vi "Read Statistics.vi"(6 "Maximum Time (10000 ms)":u32=10000, 7 "Data Source (0: Data Trace)":u16(ring) items=["Data Trace", "Memory Trace"], 8 "error in (no error)":errorcluster, 9 "Select Trace (1: 1)":u16(ring)=1 items=["1"=1, "2"=2, "3"=3, "4"=4, "5"=5, "6"=6, "7"=7, "8"=8], 10 "Measurement Type (6: Phase Noise)":u16(ring)=6 items=["AM Noise"=1, "Baseband Noise"=2, "Freq/Power"=3, "Spectrum"=4, "Transient"=5, "Phase Noise"=6, "User"=7], 11 "VISA resource name":refnum<visa-resource-name>) -> (0 "error out":errorcluster, 1 "Peak To Peak":dbl format="%^#_9g", 2 "Standard Deviation":dbl format="%^#_9g", 3 "VISA resource name out":refnum<visa-resource-name>, 5 "Mean":dbl format="%^#_9g")   [LabVIEW 2011, in "Agilent E5052X.lvlib"]
doc: "Reads the Mean, Standard Deviation and Peak To Peak values of either data or memory trace measurements of any measurement."
uses:
  Agilent E5052X.lvlib
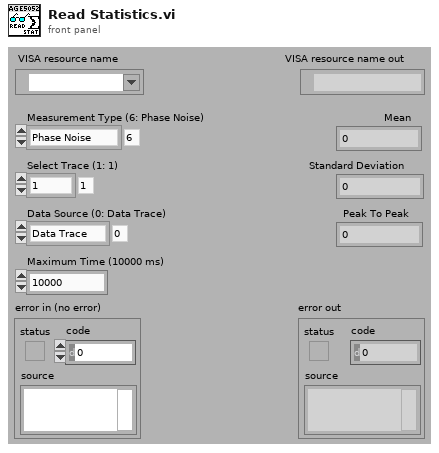
[diagram p1: front panel]
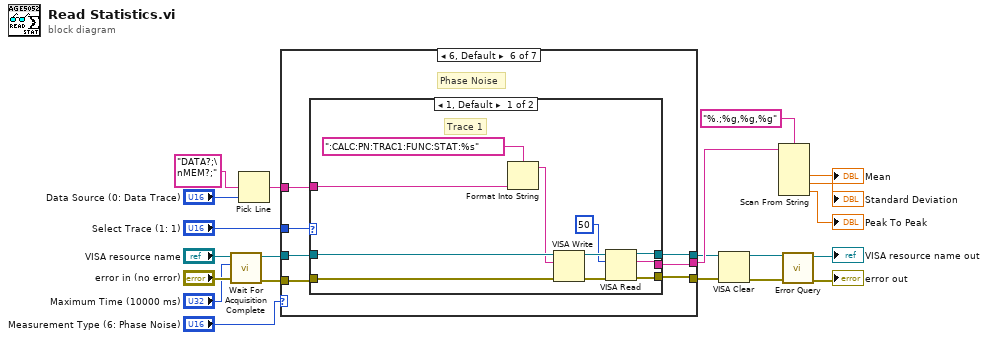
[diagram p0: block diagram]
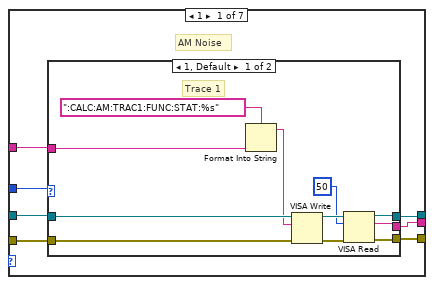
[diagram p2: hidden frame]
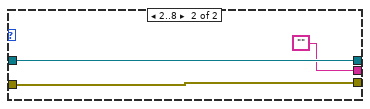
[diagram p3: hidden frame]
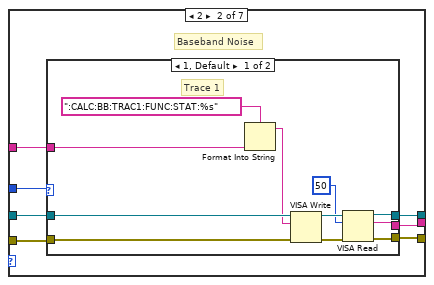
[diagram p4: hidden frame]
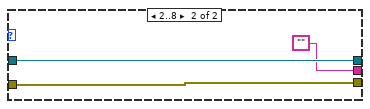
[diagram p5: hidden frame]
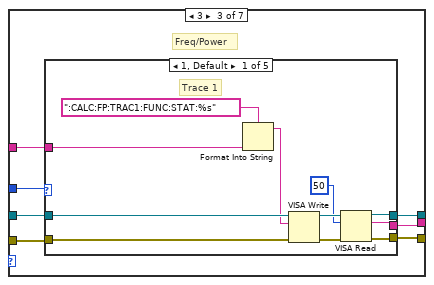
[diagram p6: hidden frame]
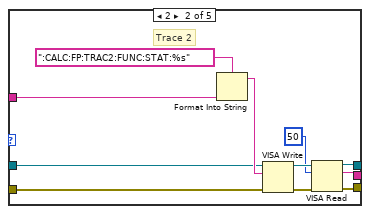
[diagram p7: hidden frame]
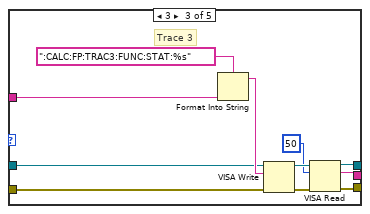
[diagram p8: hidden frame]
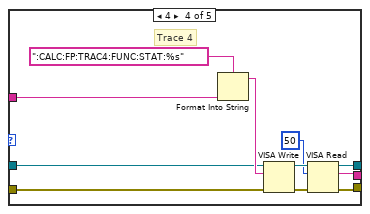
[diagram p9: hidden frame]
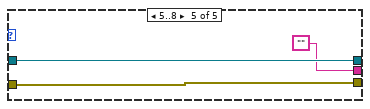
[diagram p10: hidden frame]
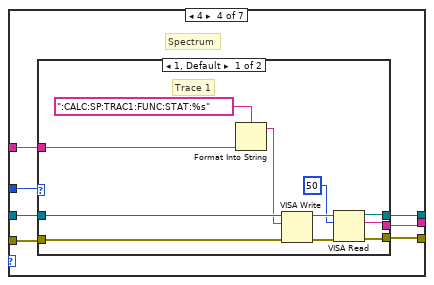
[diagram p11: hidden frame]
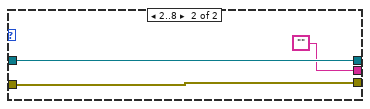
[diagram p12: hidden frame]
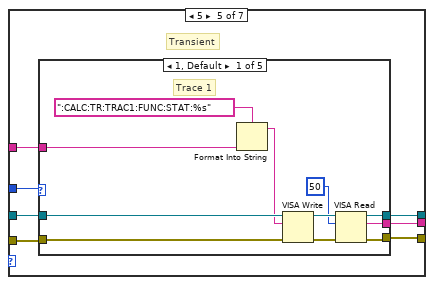
[diagram p13: hidden frame]
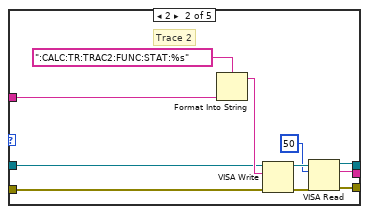
[diagram p14: hidden frame]
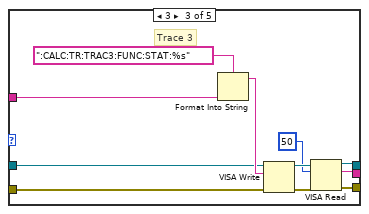
[diagram p15: hidden frame]
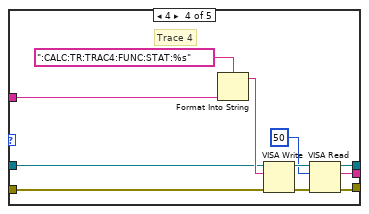
[diagram p16: hidden frame]
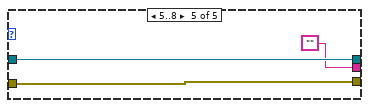
[diagram p17: hidden frame]
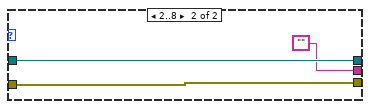
[diagram p18: hidden frame]
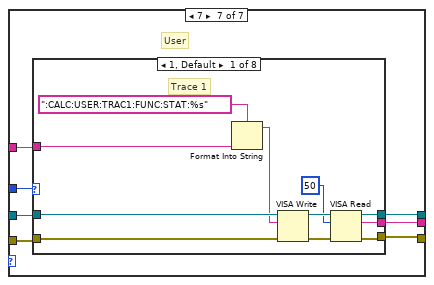
[diagram p19: hidden frame]
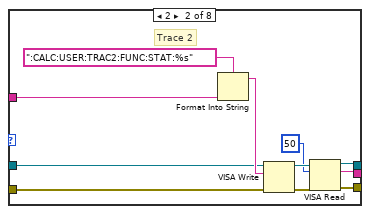
[diagram p20: hidden frame]
diagram:
  n1 = call "Wait For Acquisition Complete.vi"("error in (no error)"="error in (no error)", "Maximum Time (10000)"="Maximum Time (10000 ms)", "VISA resource name"="VISA resource name") -> ("error out"=w6:errorcluster, "VISA resource name out"=w7:refnum<visa-resource-name>)  [unwired: 7 in]
  n2 = Pick Line(multi-line string="DATA?;\nMEM?;", line index="Data Source (0: Data Trace)") -> (output string=w8:string)  [unwired: 1 in]
  n3 = case shown="6, Default" "Measurement Type (6: Phase Noise)" {
    tunnel: w6 -> [w25 w46 w67 w121 w142 w196 w217]
    tunnel: w7 -> [w26 w47 w68 w122 w143 w197 w218]
    tunnel: w8 -> [w28 w49 w69 w124 w145 w199 w220]
    tunnel: "Select Trace (1: 1)" -> [w27 w48 w70 w123 w144 w198 w219]
    tunnel: [w24 w45 w66 w120 w141 w194 w216] -> w15
    tunnel: [w22 w44 w65 w118 w140 w193 w214] -> w14
    tunnel: [w23 w43 w64 w119 w139 w195 w215] -> w19
    frame 1 {
      # "AM Noise"
      n4 = case shown="1, Default" w27 {
        tunnel: w28 -> [w39 _]
        tunnel: w26 -> [w37 w42]
        tunnel: w25 -> [w36 w41]
        tunnel: [w31 w42] -> w24
        tunnel: [w30 w41] -> w22
        tunnel: [w29 ""] -> w23
        frame 1, Default {
          # "Trace 1"
          n5 = Format Into String(format string=":CALC:AM:TRAC1:FUNC:STAT:%s", w39) -> (resulting string=w35:string)  [unwired: 2 in, 1 out]
          n6 = VISA Write(VISA resource name=w37, write buffer=w35, error in (no error)=w36) -> (VISA resource name out=w34:refnum<visa-resource-name>, error out=w33:errorcluster)  [unwired: 1 out]
          n7 = VISA Read(VISA resource name=w34, byte count=u32 50, error in (no error)=w33) -> (VISA resource name out=w31:refnum<visa-resource-name>, read buffer=w29:string, error out=w30:errorcluster)  [unwired: 1 out]
        }
        frame 2..8 {
        }
      }
    }
    frame 2 {
      # "Baseband Noise"
      n8 = case shown="1, Default" w48 {
        tunnel: w49 -> [w60 _]
        tunnel: w47 -> [w58 w63]
        tunnel: w46 -> [w57 w62]
        tunnel: [w52 w63] -> w45
        tunnel: [w51 w62] -> w44
        tunnel: [w50 ""] -> w43
        frame 1, Default {
          # "Trace 1"
          n9 = Format Into String(format string=":CALC:BB:TRAC1:FUNC:STAT:%s", w60) -> (resulting string=w56:string)  [unwired: 2 in, 1 out]
          n10 = VISA Write(VISA resource name=w58, write buffer=w56, error in (no error)=w57) -> (VISA resource name out=w55:refnum<visa-resource-name>, error out=w54:errorcluster)  [unwired: 1 out]
          n11 = VISA Read(VISA resource name=w55, byte count=u32 50, error in (no error)=w54) -> (VISA resource name out=w52:refnum<visa-resource-name>, read buffer=w50:string, error out=w51:errorcluster)  [unwired: 1 out]
        }
        frame 2..8 {
        }
      }
    }
    frame 3 {
      # "Freq/Power"
      n12 = case shown="1, Default" w70 {
        tunnel: w69 -> [w81 w90 w101 w112 _]
        tunnel: w68 -> [w79 w89 w100 w111 w117]
        tunnel: w67 -> [w78 w88 w99 w110 w116]
        tunnel: [w73 w85 w95 w107 w117] -> w66
        tunnel: [w72 w84 w98 w106 w116] -> w65
        tunnel: [w71 w82 w93 w105 ""] -> w64
        frame 1, Default {
          # "Trace 1"
          n13 = Format Into String(format string=":CALC:FP:TRAC1:FUNC:STAT:%s", w81) -> (resulting string=w77:string)  [unwired: 2 in, 1 out]
          n14 = VISA Write(VISA resource name=w79, write buffer=w77, error in (no error)=w78) -> (VISA resource name out=w76:refnum<visa-resource-name>, error out=w75:errorcluster)  [unwired: 1 out]
          n15 = VISA Read(VISA resource name=w76, byte count=u32 50, error in (no error)=w75) -> (VISA resource name out=w73:refnum<visa-resource-name>, read buffer=w71:string, error out=w72:errorcluster)  [unwired: 1 out]
        }
        frame 2 {
          # "Trace 2"
          n16 = Format Into String(format string=":CALC:FP:TRAC2:FUNC:STAT:%s", w90) -> (resulting string=w91:string)  [unwired: 2 in, 1 out]
          n17 = VISA Write(VISA resource name=w89, write buffer=w91, error in (no error)=w88) -> (VISA resource name out=w87:refnum<visa-resource-name>, error out=w86:errorcluster)  [unwired: 1 out]
          n18 = VISA Read(VISA resource name=w87, byte count=u32 50, error in (no error)=w86) -> (VISA resource name out=w85:refnum<visa-resource-name>, read buffer=w82:string, error out=w84:errorcluster)  [unwired: 1 out]
        }
        frame 3 {
          # "Trace 3"
          n19 = Format Into String(format string=":CALC:FP:TRAC3:FUNC:STAT:%s", w101) -> (resulting string=w102:string)  [unwired: 2 in, 1 out]
          n20 = VISA Write(VISA resource name=w100, write buffer=w102, error in (no error)=w99) -> (VISA resource name out=w97:refnum<visa-resource-name>, error out=w96:errorcluster)  [unwired: 1 out]
          n21 = VISA Read(VISA resource name=w97, byte count=u32 50, error in (no error)=w96) -> (VISA resource name out=w95:refnum<visa-resource-name>, read buffer=w93:string, error out=w98:errorcluster)  [unwired: 1 out]
        }
        frame 4 {
          # "Trace 4"
          n22 = Format Into String(format string=":CALC:FP:TRAC4:FUNC:STAT:%s", w112) -> (resulting string=w113:string)  [unwired: 2 in, 1 out]
          n23 = VISA Write(VISA resource name=w111, write buffer=w113, error in (no error)=w110) -> (VISA resource name out=w109:refnum<visa-resource-name>, error out=w108:errorcluster)  [unwired: 1 out]
          n24 = VISA Read(VISA resource name=w109, byte count=u32 50, error in (no error)=w108) -> (VISA resource name out=w107:refnum<visa-resource-name>, read buffer=w105:string, error out=w106:errorcluster)  [unwired: 1 out]
        }
        frame 5..8 {
        }
      }
    }
    frame 4 {
      # "Spectrum"
      n25 = case shown="1, Default" w123 {
        tunnel: w124 -> [w135 _]
        tunnel: w122 -> [w133 w138]
        tunnel: w121 -> [w132 w137]
        tunnel: [w127 w138] -> w120
        tunnel: [w126 w137] -> w118
        tunnel: [w125 ""] -> w119
        frame 1, Default {
          # "Trace 1"
          n26 = Format Into String(format string=":CALC:SP:TRAC1:FUNC:STAT:%s", w135) -> (resulting string=w131:string)  [unwired: 2 in, 1 out]
          n27 = VISA Write(VISA resource name=w133, write buffer=w131, error in (no error)=w132) -> (VISA resource name out=w130:refnum<visa-resource-name>, error out=w129:errorcluster)  [unwired: 1 out]
          n28 = VISA Read(VISA resource name=w130, byte count=u32 50, error in (no error)=w129) -> (VISA resource name out=w127:refnum<visa-resource-name>, read buffer=w125:string, error out=w126:errorcluster)  [unwired: 1 out]
        }
        frame 2..8 {
        }
      }
    }
    frame 5 {
      # "Transient"
      n29 = case shown="1, Default" w144 {
        tunnel: w145 -> [w156 w165 w176 w187 _]
        tunnel: w143 -> [w154 w164 w175 w186 w192]
        tunnel: w142 -> [w153 w163 w174 w185 w191]
        tunnel: [w148 w159 w170 w183 w192] -> w141
        tunnel: [w147 w162 w173 w182 w191] -> w140
        tunnel: [w146 w158 w168 w184 ""] -> w139
        frame 1, Default {
          # "Trace 1"
          n30 = Format Into String(format string=":CALC:TR:TRAC1:FUNC:STAT:%s", w156) -> (resulting string=w152:string)  [unwired: 2 in, 1 out]
          n31 = VISA Write(VISA resource name=w154, write buffer=w152, error in (no error)=w153) -> (VISA resource name out=w150:refnum<visa-resource-name>, error out=w151:errorcluster)  [unwired: 1 out]
          n32 = VISA Read(VISA resource name=w150, byte count=u32 50, error in (no error)=w151) -> (VISA resource name out=w148:refnum<visa-resource-name>, read buffer=w146:string, error out=w147:errorcluster)  [unwired: 1 out]
        }
        frame 2 {
          # "Trace 2"
          n33 = Format Into String(format string=":CALC:TR:TRAC2:FUNC:STAT:%s", w165) -> (resulting string=w166:string)  [unwired: 2 in, 1 out]
          n34 = VISA Write(VISA resource name=w164, write buffer=w166, error in (no error)=w163) -> (VISA resource name out=w161:refnum<visa-resource-name>, error out=w160:errorcluster)  [unwired: 1 out]
          n35 = VISA Read(VISA resource name=w161, byte count=u32 50, error in (no error)=w160) -> (VISA resource name out=w159:refnum<visa-resource-name>, read buffer=w158:string, error out=w162:errorcluster)  [unwired: 1 out]
        }
        frame 3 {
          # "Trace 3"
          n36 = Format Into String(format string=":CALC:TR:TRAC3:FUNC:STAT:%s", w176) -> (resulting string=w177:string)  [unwired: 2 in, 1 out]
          n37 = VISA Write(VISA resource name=w175, write buffer=w177, error in (no error)=w174) -> (VISA resource name out=w172:refnum<visa-resource-name>, error out=w171:errorcluster)  [unwired: 1 out]
          n38 = VISA Read(VISA resource name=w172, byte count=u32 50, error in (no error)=w171) -> (VISA resource name out=w170:refnum<visa-resource-name>, read buffer=w168:string, error out=w173:errorcluster)  [unwired: 1 out]
        }
        frame 4 {
          # "Trace 4"
          n39 = Format Into String(format string=":CALC:TR:TRAC4:FUNC:STAT:%s", w187) -> (resulting string=w188:string)  [unwired: 2 in, 1 out]
          n40 = VISA Write(VISA resource name=w186, write buffer=w188, error in (no error)=w185) -> (VISA resource name out=w180:refnum<visa-resource-name>, error out=w181:errorcluster)  [unwired: 1 out]
          n41 = VISA Read(VISA resource name=w180, byte count=u32 50, error in (no error)=w181) -> (VISA resource name out=w183:refnum<visa-resource-name>, read buffer=w184:string, error out=w182:errorcluster)  [unwired: 1 out]
        }
        frame 5..8 {
        }
      }
    }
    frame 6, Default {
      # "Phase Noise"
      n42 = case shown="1, Default" w198 {
        tunnel: w199 -> [w210 _]
        tunnel: w197 -> [w208 w213]
        tunnel: w196 -> [w207 w212]
        tunnel: [w202 w213] -> w194
        tunnel: [w201 w212] -> w193
        tunnel: [w200 ""] -> w195
        frame 1, Default {
          # "Trace 1"
          n43 = Format Into String(format string=":CALC:PN:TRAC1:FUNC:STAT:%s", w210) -> (resulting string=w206:string)  [unwired: 2 in, 1 out]
          n44 = VISA Write(VISA resource name=w208, write buffer=w206, error in (no error)=w207) -> (VISA resource name out=w205:refnum<visa-resource-name>, error out=w204:errorcluster)  [unwired: 1 out]
          n45 = VISA Read(VISA resource name=w205, byte count=u32 50, error in (no error)=w204) -> (VISA resource name out=w202:refnum<visa-resource-name>, read buffer=w200:string, error out=w201:errorcluster)  [unwired: 1 out]
        }
        frame 2..8 {
        }
      }
    }
    frame 7 {
      # "User"
      n46 = case shown="1, Default" w219 {
        tunnel: w220 -> [w231 w240 w251 w262 w270 w281 w292 w303]
        tunnel: w218 -> [w229 w239 w250 w261 w269 w280 w291 w302]
        tunnel: w217 -> [w228 w238 w249 w260 w268 w279 w290 w301]
        tunnel: [w223 w234 w245 w258 w267 w278 w289 w300] -> w216
        tunnel: [w222 w237 w248 w257 w266 w277 w288 w299] -> w214
        tunnel: [w221 w233 w243 w259 w265 w276 w287 w298] -> w215
        frame 1, Default {
          # "Trace 1"
          n47 = Format Into String(format string=":CALC:USER:TRAC1:FUNC:STAT:%s", w231) -> (resulting string=w227:string)  [unwired: 2 in, 1 out]
          n48 = VISA Write(VISA resource name=w229, write buffer=w227, error in (no error)=w228) -> (VISA resource name out=w225:refnum<visa-resource-name>, error out=w226:errorcluster)  [unwired: 1 out]
          n49 = VISA Read(VISA resource name=w225, byte count=u32 50, error in (no error)=w226) -> (VISA resource name out=w223:refnum<visa-resource-name>, read buffer=w221:string, error out=w222:errorcluster)  [unwired: 1 out]
        }
        frame 2 {
          # "Trace 2"
          n50 = Format Into String(format string=":CALC:USER:TRAC2:FUNC:STAT:%s", w240) -> (resulting string=w241:string)  [unwired: 2 in, 1 out]
          n51 = VISA Write(VISA resource name=w239, write buffer=w241, error in (no error)=w238) -> (VISA resource name out=w236:refnum<visa-resource-name>, error out=w235:errorcluster)  [unwired: 1 out]
          n52 = VISA Read(VISA resource name=w236, byte count=u32 50, error in (no error)=w235) -> (VISA resource name out=w234:refnum<visa-resource-name>, read buffer=w233:string, error out=w237:errorcluster)  [unwired: 1 out]
        }
        frame 3 {
          # "Trace 3"
          n53 = Format Into String(format string=":CALC:USER:TRAC3:FUNC:STAT:%s", w251) -> (resulting string=w252:string)  [unwired: 2 in, 1 out]
          n54 = VISA Write(VISA resource name=w250, write buffer=w252, error in (no error)=w249) -> (VISA resource name out=w247:refnum<visa-resource-name>, error out=w246:errorcluster)  [unwired: 1 out]
          n55 = VISA Read(VISA resource name=w247, byte count=u32 50, error in (no error)=w246) -> (VISA resource name out=w245:refnum<visa-resource-name>, read buffer=w243:string, error out=w248:errorcluster)  [unwired: 1 out]
        }
        frame 4 {
          # "Trace 4"
          n56 = Format Into String(format string=":CALC:USER:TRAC4:FUNC:STAT:%s", w262) -> (resulting string=w263:string)  [unwired: 2 in, 1 out]
          n57 = VISA Write(VISA resource name=w261, write buffer=w263, error in (no error)=w260) -> (VISA resource name out=w255:refnum<visa-resource-name>, error out=w256:errorcluster)  [unwired: 1 out]
          n58 = VISA Read(VISA resource name=w255, byte count=u32 50, error in (no error)=w256) -> (VISA resource name out=w258:refnum<visa-resource-name>, read buffer=w259:string, error out=w257:errorcluster)  [unwired: 1 out]
        }
        frame 5 {
          # "Trace 5"
          n59 = Format Into String(format string=":CALC:USER:TRAC5:FUNC:STAT:%s", w270) -> (resulting string=w274:string)  [unwired: 2 in, 1 out]
          n60 = VISA Write(VISA resource name=w269, write buffer=w274, error in (no error)=w268) -> (VISA resource name out=w272:refnum<visa-resource-name>, error out=w273:errorcluster)  [unwired: 1 out]
          n61 = VISA Read(VISA resource name=w272, byte count=u32 50, error in (no error)=w273) -> (VISA resource name out=w267:refnum<visa-resource-name>, read buffer=w265:string, error out=w266:errorcluster)  [unwired: 1 out]
        }
        frame 6 {
          # "Trace 6"
          n62 = Format Into String(format string=":CALC:USER:TRAC6:FUNC:STAT:%s", w281) -> (resulting string=w285:string)  [unwired: 2 in, 1 out]
          n63 = VISA Write(VISA resource name=w280, write buffer=w285, error in (no error)=w279) -> (VISA resource name out=w283:refnum<visa-resource-name>, error out=w284:errorcluster)  [unwired: 1 out]
          n64 = VISA Read(VISA resource name=w283, byte count=u32 50, error in (no error)=w284) -> (VISA resource name out=w278:refnum<visa-resource-name>, read buffer=w276:string, error out=w277:errorcluster)  [unwired: 1 out]
        }
        frame 7 {
          # "Trace 7"
          n65 = Format Into String(format string=":CALC:USER:TRAC7:FUNC:STAT:%s", w292) -> (resulting string=w296:string)  [unwired: 2 in, 1 out]
          n66 = VISA Write(VISA resource name=w291, write buffer=w296, error in (no error)=w290) -> (VISA resource name out=w294:refnum<visa-resource-name>, error out=w295:errorcluster)  [unwired: 1 out]
          n67 = VISA Read(VISA resource name=w294, byte count=u32 50, error in (no error)=w295) -> (VISA resource name out=w289:refnum<visa-resource-name>, read buffer=w287:string, error out=w288:errorcluster)  [unwired: 1 out]
        }
        frame 8 {
          # "Trace 8"
          n68 = Format Into String(format string=":CALC:USER:TRAC8:FUNC:STAT:%s", w303) -> (resulting string=w307:string)  [unwired: 2 in, 1 out]
          n69 = VISA Write(VISA resource name=w302, write buffer=w307, error in (no error)=w301) -> (VISA resource name out=w305:refnum<visa-resource-name>, error out=w306:errorcluster)  [unwired: 1 out]
          n70 = VISA Read(VISA resource name=w305, byte count=u32 50, error in (no error)=w306) -> (VISA resource name out=w300:refnum<visa-resource-name>, read buffer=w298:string, error out=w299:errorcluster)  [unwired: 1 out]
        }
      }
    }
  }
  n71 = VISA Clear(VISA resource name=w15, error in (no error)=w14) -> (VISA resource name out=w2:refnum<visa-resource-name>, error out=w1:errorcluster)
  n72 = Scan From String(format string="%.;%g,%g,%g", input string=w19) -> (output 1=→"Mean":dbl, output 2=→"Standard Deviation":dbl, output 3=→"Peak To Peak":dbl)  [unwired: 5 in, 3 out]
  n73 = call "Error Query.vi"("error in (no error)"=w1, "VISA resource name"=w2) -> ("error out"=→"error out":errorcluster, "VISA resource name out"=→"VISA resource name out":refnum<visa-resource-name>)  [unwired: 6 in, 2 out]
